vi "test.vi"() -> ()   [LabVIEW 2010, in "Image.lvclass"]
uses:
  Image.lvclass
  storage_mode.ctl
  clusters/pixel_coordinate_cluster.ctl
  insert_mode_enum.ctl
  clusters/calibration.ctl
  enumerations/unit.ctl
  target_format_enum.ctl
panel:
  in  "Image Type":T1 items=["Grayscale (U8)", "Grayscale (I16)", "Grayscale (SGL)", "Complex (CSG)", "RGB (U32)", "HSL (U32)", "RGB (U64)", "Grayscale (U16)"]
  in  "Tab Control":T2(tab)
  in  "load":bool
  in  "write binary file":bool
  in  "save":bool
  in  "load from binary":bool
  in  "force format?":T3
  in  "add":bool
  in  "subtract":bool
  in  "divide":bool
  in  "divisor":dbl=1.0
  in  "offset and range":bool
  in  "offset":dbl
  in  "range":dbl
  in  "multiply":bool
  in  "factor":dbl=1.0
  in  "divide by image":bool
  in  "expression":string
  in  "evaluate expression":bool
  in  "number of images":i32
  in  "colour values above?":bool
  in  "colour values below?":bool
  in  "rotate":bool
  in  "downsample":bool
  in  "x factor":dbl=2.0 min=1.0
  in  "y factor":dbl=2.0 min=1.0
  in  "scale to max":bool
  in  "max side length":i32
  in  "angle":dbl[unit]
  in  "clear":bool
  in  "random fill":bool
  in  "insert block":bool
  in  "pixel coordinate":T4
  in  "mode":T5
  in  "repetition":i32=1 min=1
  in  "enable scale bar":bool
  in  "calibration":T6={"x"=1.0, "y"=1.0, "z"=0.0, "x unit"=enum."um", "y unit"=enum."um", "z unit"=enum."um"}
  in  "enable x middle line?":bool
  in  "enable y middle line?":bool
  in  "storage type":T8
  in  "stop":bool
  out "Image":T9(plugin-control)
  # "Test Image"
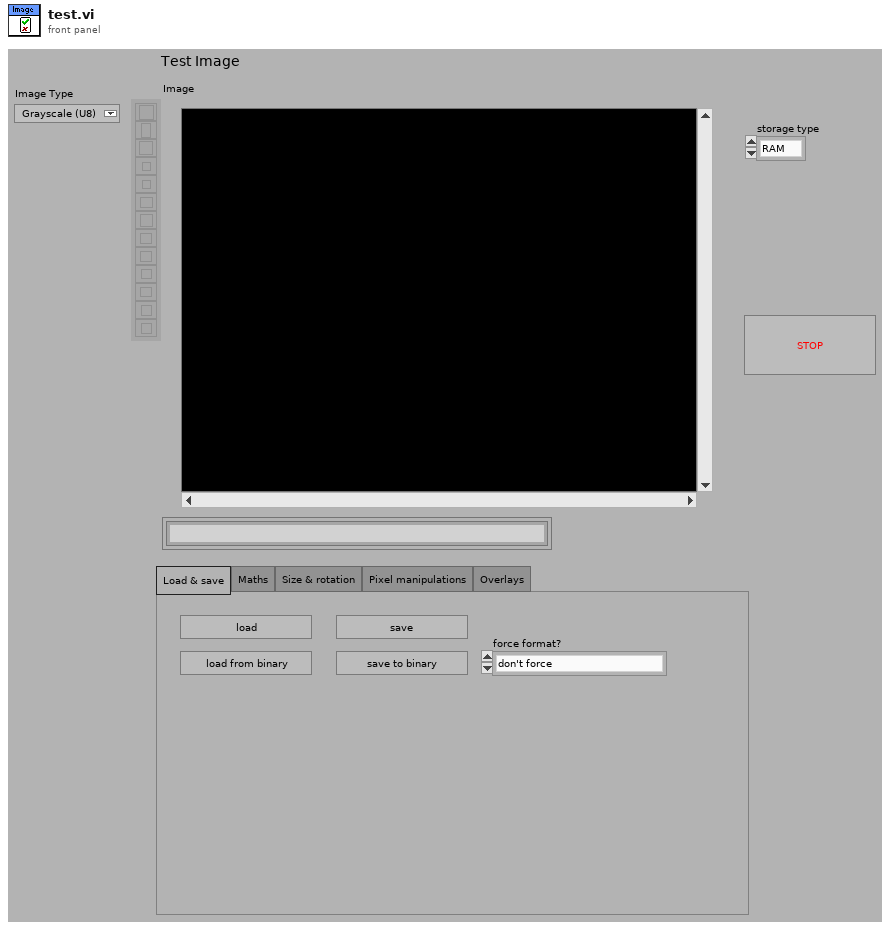
[diagram p1: front panel]
types:
  T1 = typedef "Image Type" = u32
  T2 = enum32{"Load & save", "Maths", "Size & rotation", "Pixel manipulations", "Overlays"}
  T3 = typedef "target_format_enum.ctl" = enum16{"don't force", "uint8", "uint16", "int16", "uint32", "int32", "single float"}
  T4 = typedef "pixel_coordinate_cluster.ctl" = cluster{"x":i32, "y":i32}
  T5 = typedef "Image.lvclass/insert_mode_enum.ctl" = enum16{"replace", "average"}
  T6 = typedef "calibration.ctl" = cluster{"x":dbl, "y":dbl, "z":dbl, "x unit":T7, "y unit":T7, "z unit":T7}
  T7 = typedef "Image.lvclass/unit.ctl" = enum16{"um", "s"}
  T8 = typedef "Image.lvclass/storage_mode.ctl" = enum16{"RAM", "disk"}
  T9 = typedef "IMAQ Image.ctl" = refnum<image>
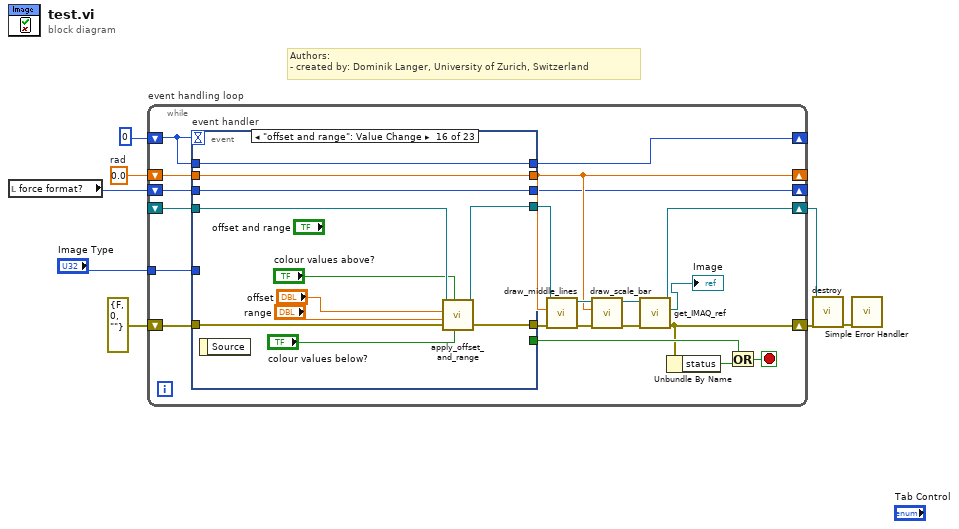
[diagram p0: block diagram]
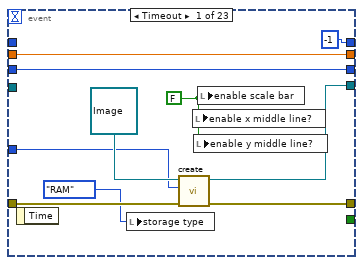
[diagram p2: hidden frame]
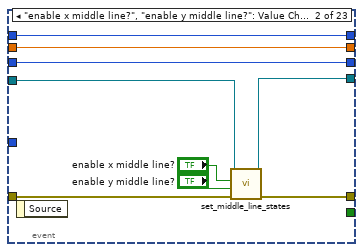
[diagram p3: hidden frame]
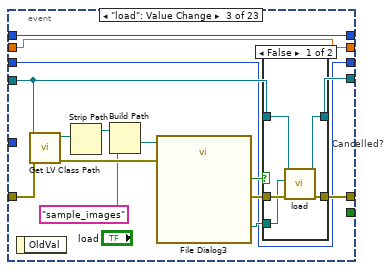
[diagram p4: hidden frame]
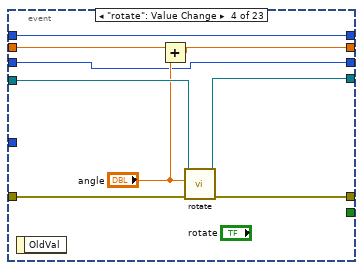
[diagram p6: hidden frame]
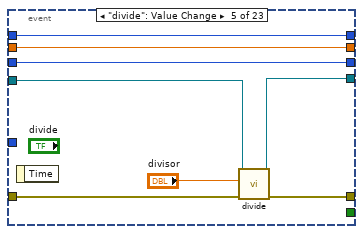
[diagram p7: hidden frame]
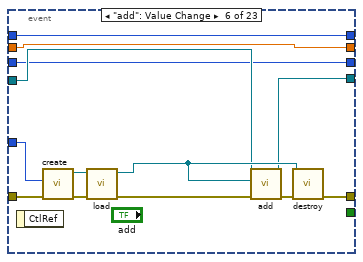
[diagram p8: hidden frame]
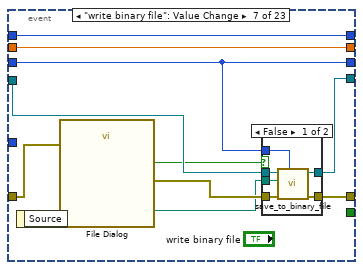
[diagram p9: hidden frame]
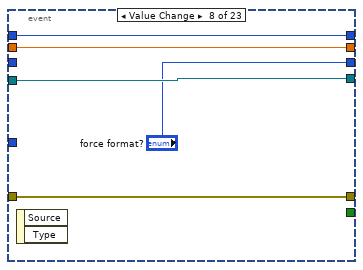
[diagram p11: hidden frame]
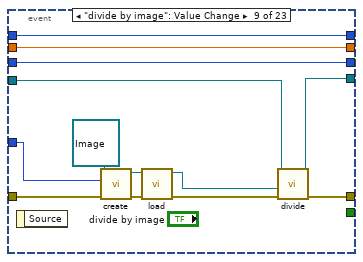
[diagram p12: hidden frame]
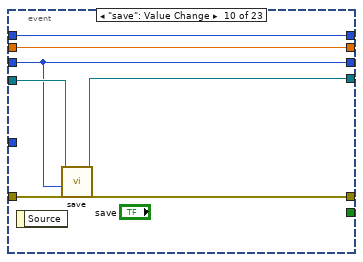
[diagram p13: hidden frame]
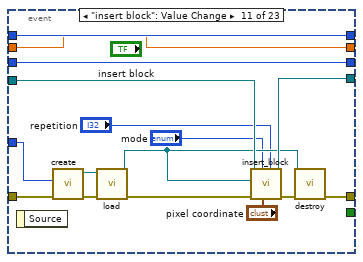
[diagram p14: hidden frame]
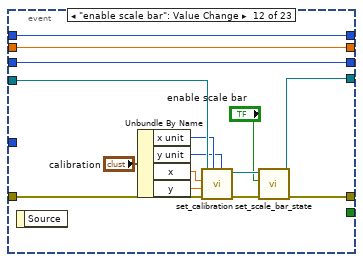
[diagram p15: hidden frame]
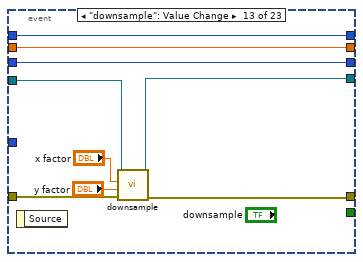
[diagram p16: hidden frame]
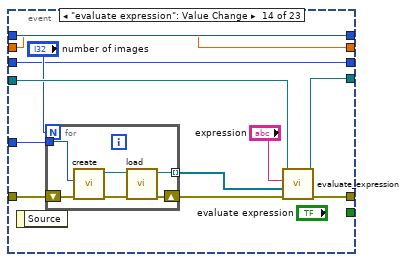
[diagram p17: hidden frame]
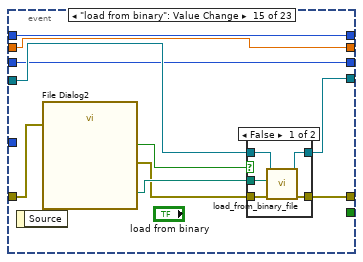
[diagram p18: hidden frame]
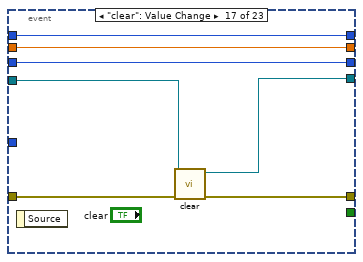
[diagram p20: hidden frame]
diagram:
  w3 = dbl[unit] 0.0  # rad
  # "Authors: \n- created by: Dominik Langer, University of Zurich, Switzerland"
  n1 = local read "force format?"() -> (w1:T3)
  n2 = while "event handling loop" {
    shift-right: [w25] -> w7
    shift-left: _ -> [w29]
    shift-right: [w27] -> _
    shift-left: 0 -> [w28]
    shift-right: [w9] -> w6
    shift-left: errorcluster {"status"=FALSE, "code"=0, "source"=""} ("error out") -> [w26]
    tunnel: "Image Type" -> [w21]
    shift-right: [w13] -> _
    shift-left: w3 -> [w18]
    shift-right: [w12] -> _
    shift-left: w1 -> [w11]
    stop <- w23 stop-if-true
    n3 = event "event handler" shown="[15] \"offset and range\": Value Change" {
      selector: _ -> [_ _ _ _ _ _ _ _ _ _ _ _ _ _ _ _ _ _ _ _ _ _ _]
      dyn-events: _ -> [_ _ _ _ _ _ _ _ _ _ _ _ _ _ _ _ _ _ _ _ _ _ _]
      timeout: w28 -> [_ _ _ _ _ _ _ _ _ _ _ _ _ _ _ _ _ _ _ _ _ _ _]
      tunnel: [w39 w44 w62 w75 w84 w90 w104 w123 w129 w139 w157 w165 w180 w192 w205 w227 w233 w241 w250 w258 w267 w273 w288] -> w19
      tunnel: w29 -> [_ w45 w55 w76 w85 w91 w107 w123 w127 w140 w158 w172 w181 w193 w207 w228 w234 w242 w251 w259 w268 w274 w288]
      tunnel: w28 -> [_ w48 w63 w79 w82 w98 w103 w122 w126 w143 w159 w174 w178 w195 w204 w229 w232 w240 w249 w256 w266 w275 w287]
      tunnel: [-1 w48 w63 w79 w82 w98 w103 w122 w126 w143 w159 w174 w178 w195 w204 w229 w232 w240 w249 w256 w266 w275 w287] -> w27
      tunnel: [w37 w46 w61 w77 w86 w96 w110 w121 w130 w141 w150 w167 w182 w194 w208 w219 w235 w243 w252 w257 w265 w276 w289] -> w20
      tunnel: w26 -> [w36 w47 w57 w78 w87 w100 w109 w121 w131 w142 w154 w173 w183 w190 w211 w220 w236 w244 w253 w261 w269 w278 w289]
      tunnel: [_ _ _ _ _ _ _ _ _ _ _ _ _ _ _ _ _ _ _ _ _ _ TRUE] -> w22
      tunnel: w21 -> [w31 _ _ _ _ w99 _ _ w128 _ w152 _ _ w188 _ _ _ _ _ _ _ w272 _]
      tunnel: w18 -> [w32 w41 w50 w73 w81 w89 w102 w120 w125 w138 w145 w161 w176 w185 w203 w224 w231 w238 w246 w255 w263 w271 w285]
      tunnel: [w32 w41 w50 w72 w81 w89 w102 w120 w125 w138 w145 w161 w176 w185 w203 w224 w231 w238 w246 w255 w263 w271 w285] -> w13
      tunnel: [w30 w40 w49 w71 w80 w88 w101 "force format?" w124 w137 w144 w160 w175 w184 w202 w223 w230 w237 w245 w254 w262 w270 w284] -> w12
      tunnel: w11 -> [w30 w40 w49 w71 w80 w88 w101 _ w124 w137 w144 w160 w175 w184 w202 w223 w230 w237 w245 w254 w262 w270 w284]
      event Timeout {
        w33 = FALSE
        n4 = event-data() -> ()  [unwired: 2 out]
        n5 = local write "storage type"(storage_mode."RAM" ("storage type")) -> ()
        n6 = call "create.vi"("error in (no error)"=w36, "Image Type"=w31, "Image in"=refnum<class "Image.lvclass"> refnum ("Image.lvclass")) -> ("error out"=w37:errorcluster, "Image out"=w39:refnum<class "Image.lvclass">)  [unwired: 1 in, 6 out]
        n7 = local write "enable x middle line?"(w33) -> ()
        n8 = local write "enable y middle line?"(w33) -> ()
        n9 = local write "enable scale bar"(w33) -> ()
      }
      event "enable x middle line?", "enable y middle line?": Value Change {
        n10 = event-data() -> ()  [unwired: 2 out]
        n11 = call "set_middle_line_states.vi"("error in (no error)"=w47, "draw y line?"="enable y middle line?", "draw x line?"="enable x middle line?", "Image in"=w45) -> ("error out"=w46:errorcluster, "Image out"=w44:refnum<class "Image.lvclass">)  [unwired: 6 out]
      }
      event "load": Value Change {
        n12 = event-data() -> ()  [unwired: 2 out]
        n13 = call <vilib>:"Get LV Class Path.vi"("error in (no error)"=w57, "object"=w55) -> ("error out"=w56:errorcluster, "class path"=w52:path)  [unwired: 8 in]
        n14 = Strip Path(path=w52) -> (stripped path=w51:path)  [unwired: 1 out]
        n15 = Build Path(base path=w51, name or relative path="sample_images") -> (appended path=w54:path)
        n16 = call "File Dialog3"("start path"=w54, "error in"=w56) -> ("selected path"=w58:path, "cancelled"=w59:bool, "error out"=w60:errorcluster)  [unwired: 10 in, 1 out]
        n17 = case "Cancelled?" shown="False" w59 {
          tunnel: [w68 w70] -> w62
          tunnel: w55 -> [w67 w70]
          tunnel: [w66 w69] -> w61
          tunnel: w60 -> [w65 w69]
          tunnel: w58 -> [w64 _]
          frame False {
            n18 = call-dynamic "load.vi"("error in (no error)"=w65, "Path"=w64, "Image in"=w67) -> ("error out"=w66:errorcluster, "Image out"=w68:refnum<class "Image.lvclass">)  [unwired: 1 in, 6 out]
          }
          frame True {
          }
        }
      }
      event "rotate": Value Change {
        n19 = event-data() -> ()  [unwired: 2 out]
        n20 = Add(x=w73, y="angle") -> (x+y=w72:dbl[unit])
        n21 = call "rotate.vi"("error in (no error)"=w78, "angle"="angle", "Image in"=w76) -> ("error out"=w77:errorcluster, "Image out"=w75:refnum<class "Image.lvclass">)  [unwired: 7 in]
      }
      event "divide": Value Change {
        n22 = event-data() -> ()  [unwired: 2 out]
        n23 = call-dynamic "divide.vi"("error in (no error)"=w87, "divisor"="divisor", "Image in"=w85) -> ("error out"=w86:errorcluster, "Image out"=w84:refnum<class "Image.lvclass">)  [unwired: 1 in, 6 out]
      }
      event "add": Value Change {
        n24 = event-data() -> ()  [unwired: 2 out]
        n25 = call "create.vi"("error in (no error)"=w100, "Image Type"=w99) -> ("error out"=w95:errorcluster, "Image out"=w94:refnum<class "Image.lvclass">)  [unwired: 2 in, 6 out]
        n26 = call-dynamic "load.vi"("error in (no error)"=w95, "Image in"=w94) -> ("error out"=w93:errorcluster, "Image out"=w92:refnum<class "Image.lvclass">)  [unwired: 2 in, 6 out]
        n27 = call-dynamic "add.vi"("error in (no error)"=w93, "addend"=w92, "Image in"=w91) -> ("error out"=w97:errorcluster, "Image out"=w90:refnum<class "Image.lvclass">)  [unwired: 1 in, 6 out]
        n28 = call-dynamic "destroy.vi"("error in (no error)"=w97, "Image in"=w92) -> ("error out"=w96:errorcluster)  [unwired: 9 out]
      }
      event "write binary file": Value Change {
        n29 = event-data() -> ()  [unwired: 2 out]
        n30 = call "File Dialog"("error in"=w109) -> ("selected path"=w106:path, "cancelled"=w105:bool, "error out"=w108:errorcluster)  [unwired: 6 in, 6 out]
        n31 = case shown="False" w105 {
          tunnel: [w116 w118] -> w110
          tunnel: w108 -> [w115 w118]
          tunnel: w107 -> [w114 w117]
          tunnel: w106 -> [w113 _]
          tunnel: [w112 w117] -> w104
          tunnel: w101 -> [w111 _]
          frame False {
            n32 = call-dynamic "save_to_binary_file.vi"("force format?"=w111, "error in (no error)"=w115, "Path"=w113, "Image in"=w114) -> ("error out"=w116:errorcluster, "Image out"=w112:refnum<class "Image.lvclass">)  [unwired: 4 in, 2 out]
          }
          frame True {
          }
        }
      }
      event Value Change {
        n33 = event-data() -> ()  [unwired: 3 out]
      }
      event "divide by image": Value Change {
        n34 = event-data() -> ()  [unwired: 2 out]
        n35 = call "create.vi"("error in (no error)"=w131, "Image Type"=w128, "Image in"=refnum<class "Image.lvclass"> refnum ("Image.lvclass")) -> ("error out"=w133:errorcluster, "Image out"=w134:refnum<class "Image.lvclass">)  [unwired: 1 in, 6 out]
        n36 = call-dynamic "load.vi"("error in (no error)"=w133, "Image in"=w134) -> ("error out"=w135:errorcluster, "Image out"=w136:refnum<class "Image.lvclass">)  [unwired: 2 in, 6 out]
        n37 = call-dynamic "divide.vi"("error in (no error)"=w135, "divisor"=w136, "Image in"=w127) -> ("error out"=w130:errorcluster, "Image out"=w129:refnum<class "Image.lvclass">)  [unwired: 1 in, 6 out]
      }
      event "save": Value Change {
        n38 = event-data() -> ()  [unwired: 2 out]
        n39 = call "save.vi"("error in (no error)"=w142, "force format?"=w137, "Image in"=w140) -> ("error out"=w141:errorcluster, "Image out"=w139:refnum<class "Image.lvclass">)  [unwired: 2 in, 5 out]
      }
      event "insert block": Value Change {
        n40 = event-data() -> ()  [unwired: 2 out]
        n41 = call "create.vi"("error in (no error)"=w154, "Image Type"=w152) -> ("error out"=w155:errorcluster, "Image out"=w156:refnum<class "Image.lvclass">)  [unwired: 2 in, 6 out]
        n42 = call-dynamic "load.vi"("error in (no error)"=w155, "Image in"=w156) -> ("error out"=w153:errorcluster, "Image out"=w149:refnum<class "Image.lvclass">)  [unwired: 2 in, 6 out]
        n43 = call-dynamic "insert_block.vi"("repetition"="repetition", "start pixel coordinate"="pixel coordinate", "mode"="mode", "error in (no error)"=w153, "block"=w149, "Image in"=w158) -> ("error out"=w151:errorcluster, "Image out"=w157:refnum<class "Image.lvclass">)  [unwired: 4 out]
        n44 = call-dynamic "destroy.vi"("error in (no error)"=w151, "Image in"=w149) -> ("error out"=w150:errorcluster)  [unwired: 9 out]
      }
      event "enable scale bar": Value Change {
        n45 = event-data() -> ()  [unwired: 2 out]
        n46 = Unbundle By Name("calibration") -> ("x unit"=w163:T7, "y unit"=w162:T7, "x"=w171:dbl, "y"=w170:dbl)
        n47 = call "set_calibration.vi"("y unit"=w162, "x unit"=w163, "error in (no error)"=w173, "y"=w170, "x"=w171, "Image in"=w172) -> ("error out"=w168:errorcluster, "Image out"=w166:refnum<class "Image.lvclass">)  [unwired: 4 out]
        n48 = call "set_scale_bar_state.vi"("error in (no error)"=w168, "enable?"="enable scale bar", "Image in"=w166) -> ("error out"=w167:errorcluster, "Image out"=w165:refnum<class "Image.lvclass">)  [unwired: 7 out]
      }
      event "downsample": Value Change {
        n49 = event-data() -> ()  [unwired: 2 out]
        n50 = call-dynamic "downsample.vi"("error in (no error)"=w183, "y factor"="y factor", "x factor"="x factor", "Image in"=w181) -> ("error out"=w182:errorcluster, "Image out"=w180:refnum<class "Image.lvclass">)  [unwired: 6 out]
      }
      event "evaluate expression": Value Change {
        n51 = event-data() -> ()  [unwired: 2 out]
        n52 = for {
          N: "number of images" -> [_]
          tunnel: w188 -> [w197]
          shift-right: [w199] -> w189
          shift-left: w190 -> [w200]
          tunnel: [w196] -> w187 mode=indexing
          n53 = call "create.vi"("error in (no error)"=w200, "Image Type"=w197) -> ("error out"=w201:errorcluster, "Image out"=w198:refnum<class "Image.lvclass">)  [unwired: 2 in, 6 out]
          n54 = call-dynamic "load.vi"("error in (no error)"=w201, "Image in"=w198) -> ("error out"=w199:errorcluster, "Image out"=w196:refnum<class "Image.lvclass">)  [unwired: 2 in, 6 out]
        }
        n55 = call "evaluate_expression.vi"("error in (no error)"=w189, "images in"=w187, "term in"="expression", "destination image in"=w193) -> ("error out"=w194:errorcluster, "result out"=w192:refnum<class "Image.lvclass">)  [unwired: 6 out]
      }
      event "load from binary": Value Change {
        n56 = event-data() -> ()  [unwired: 2 out]
        n57 = call "File Dialog2"("error in"=w211) -> ("selected path"=w210:path, "cancelled"=w206:bool, "error out"=w209:errorcluster)  [unwired: 6 in, 6 out]
        n58 = case shown="False" w206 {
          tunnel: w210 -> [w216 _]
          tunnel: w209 -> [w215 w218]
          tunnel: [w214 w218] -> w208
          tunnel: w207 -> [w213 w217]
          tunnel: [w212 w217] -> w205
          frame False {
            n59 = call-dynamic "load_from_binary_file.vi"("error in (no error)"=w215, "Path"=w216, "Image in"=w213) -> ("error out"=w214:errorcluster, "Image out"=w212:refnum<class "Image.lvclass">)  [unwired: 7 out]
          }
          frame True {
          }
        }
      }
      event "offset and range": Value Change {
        n60 = event-data() -> ()  [unwired: 2 out]
        n61 = call-dynamic "apply_offset_and_range.vi"("colour values below?"="colour values below?", "colour values above?"="colour values above?", "error in (no error)"=w220, "range"="range", "offset"="offset", "Image in"=w228) -> ("error out"=w219:errorcluster, "Image out"=w227:refnum<class "Image.lvclass">)  [unwired: 2 in, 2 out]
      }
      event "clear": Value Change {
        n62 = event-data() -> ()  [unwired: 2 out]
        n63 = call-dynamic "clear.vi"("error in (no error)"=w236, "Image in"=w234) -> ("error out"=w235:errorcluster, "Image out"=w233:refnum<class "Image.lvclass">)  [unwired: 8 out]
      }
      event "multiply": Value Change {
        n64 = event-data() -> ()  [unwired: 2 out]
        n65 = call-dynamic "multiply.vi"("error in (no error)"=w244, "factor"="factor", "Image in"=w242) -> ("error out"=w243:errorcluster, "Image out"=w241:refnum<class "Image.lvclass">)  [unwired: 1 in, 6 out]
      }
      event "random fill": Value Change {
        n66 = event-data() -> ()  [unwired: 2 out]
        n67 = call-dynamic "random_fill.vi"("error in (no error)"=w253, "minimum value"=0.0, "maximum value"=1.0, "Image in"=w251) -> ("error out"=w252:errorcluster, "Image out"=w250:refnum<class "Image.lvclass">)  [unwired: 6 out]
      }
      event "scale to max": Value Change {
        n68 = event-data() -> ()  [unwired: 2 out]
        n69 = call-dynamic "scale_to_max.vi"("error in (no error)"=w261, "max length (pixels)"="max side length", "Image in"=w259) -> ("error out"=w257:errorcluster, "Image out"=w258:refnum<class "Image.lvclass">)  [unwired: 7 out]
      }
      event Value Change {
        n70 = event-data() -> ()  [unwired: 2 out]
        n71 = call-dynamic "swap.vi"("error in (no error)"=w269, "storage type target"="storage type", "Image in"=w268) -> ("error out"=w265:errorcluster, "Image out"=w267:refnum<class "Image.lvclass">)  [unwired: 7 out]
      }
      event "subtract": Value Change {
        n72 = event-data() -> ()  [unwired: 2 out]
        n73 = call "create.vi"("error in (no error)"=w278, "Image Type"=w272, "Image in"=refnum<class "Image.lvclass"> refnum ("Image.lvclass")) -> ("error out"=w280:errorcluster, "Image out"=w281:refnum<class "Image.lvclass">)  [unwired: 1 in, 6 out]
        n74 = call-dynamic "load.vi"("error in (no error)"=w280, "Image in"=w281) -> ("error out"=w282:errorcluster, "Image out"=w283:refnum<class "Image.lvclass">)  [unwired: 2 in, 6 out]
        n75 = call-dynamic "subtract.vi"("error in (no error)"=w282, "subtrahend"=w283, "Image in"=w274) -> ("error out"=w279:errorcluster, "Image out"=w273:refnum<class "Image.lvclass">)  [unwired: 7 out]
        n76 = call-dynamic "destroy.vi"("error in (no error)"=w279, "Image in"=w283) -> ("error out"=w276:errorcluster)  [unwired: 9 out]
      }
      event "stop": Value Change {
        n77 = event-data() -> ()  [unwired: 2 out]
      }
    }
    n78 = call "draw_middle_lines.vi"("error in (no error)"=w20, "rotation angle"=w13, "Image in"=w19) -> ("error out"=w14:errorcluster, "Image out"=w17:refnum<class "Image.lvclass">)  [unwired: 7 in]
    n79 = call "draw_scale_bar.vi"("error in (no error)"=w14, "angle"=w13, "Image in"=w17) -> ("error out"=w15:errorcluster, "Image out"=w16:refnum<class "Image.lvclass">)  [unwired: 7 in]
    n80 = call-dynamic "get_IMAQ_ref.vi"("error in (no error)"=w15, "Image.lvclass in"=w16) -> ("error out"=w9:errorcluster, "Image"=→"Image":T9, "Image.lvclass out"=w25:refnum<class "Image.lvclass">)  [unwired: 7 out]
    n81 = Unbundle By Name(w9) -> ("status"=w24:bool)
    n82 = Or(x=w22, y=w24) -> (x .or. y?=w23:bool)
  }
  n83 = call-dynamic "destroy.vi"("error in (no error)"=w6, "Image in"=w7) -> ("error out"=w4:errorcluster)  [unwired: 9 out]
  n84 = call <vilib>:"Simple Error Handler.vi"("error in (no error)"=w4) -> ()  [unwired: 4 in, 5 out]
